vi "SerialWrite&ReadToArduinoLEDBlinkyExample.vi"(8 "error in (no error)":errorcluster, 10 "Text Ring":u16(ring) items=["LED_OFF", "LED_ON"], 11 "ArduinoComPort":refnum<visa-resource-name>) -> (0 "error out":errorcluster, 3 "read buffer":string)   [LabVIEW 2020]
uses:
  <vilib>/Instr/_visa.llb/VISA Configure Serial Port (Instr).vi
panel:
  in  "Send Cmd":bool
  in  "stop":bool
  # "`"
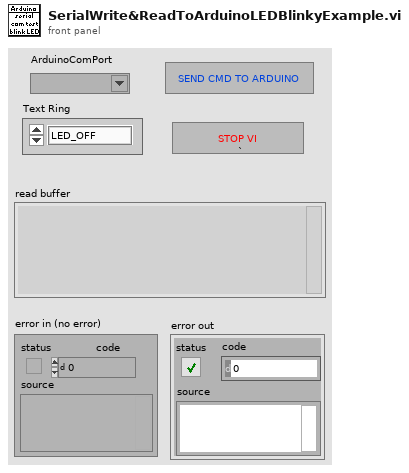
[diagram p1: front panel]
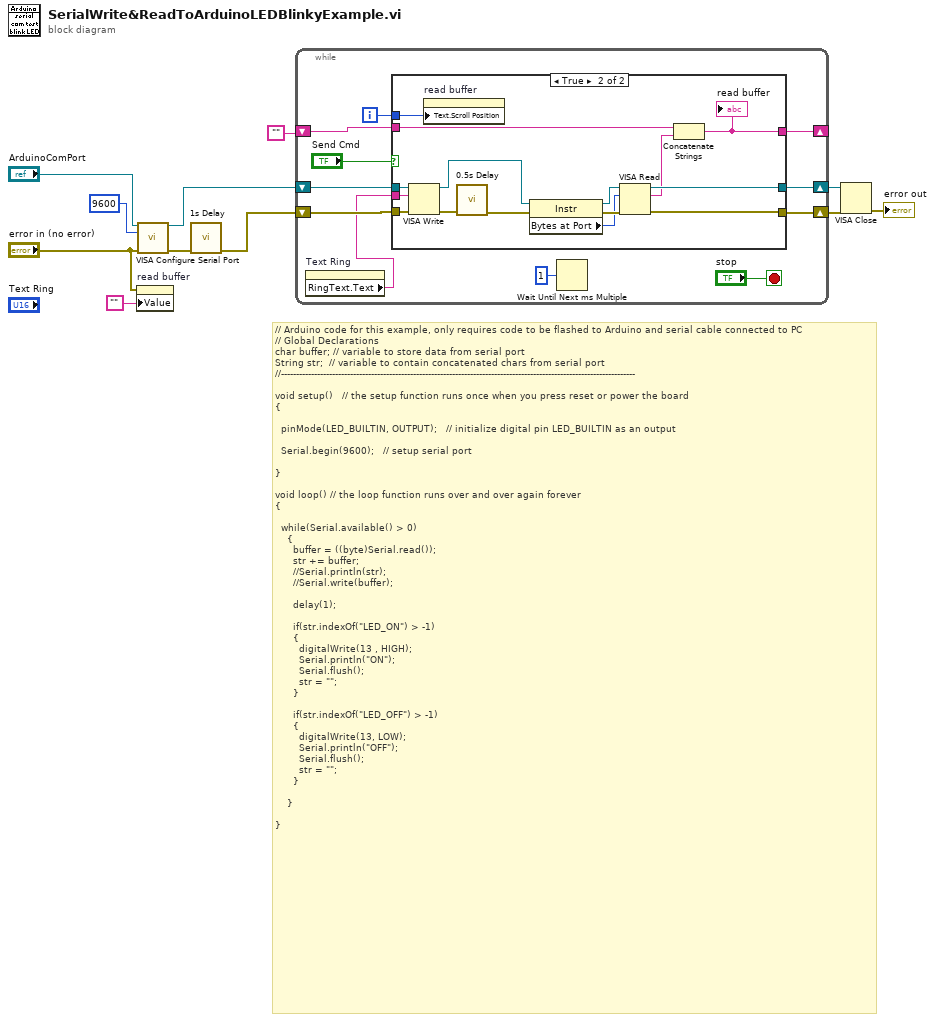
[diagram p0: block diagram]
diagram:
  # "// Arduino code for this example, only requires code to be flashed to Arduino and serial cable connected to PC\n// Global Declarations\nchar buffer; // variable to store data from serial port\nString str;  // variable to contain concatenated chars from serial port\n//----------------------------------------------------------------------------------------------------------------------\n \nvoid setup()   // the setup function runs once when you press reset or power the board \n{\n\n  pinMode(LED_BUILTIN, OUTPUT);   // initialize digital pin LED_BUILTIN as an output\n\n  Serial.begin(9600);   // setup serial port\n\n}\n\nvoid loop() // the loop function runs over and over again forever\n{\n\n  while(Serial.available() > 0)\n    {\n      buffer = ((byte)Serial.read());\n      str += buffer;\n      //Serial.println(str);\n      //Serial.write(buffer);\n\n      delay(1);\n      \n      if(str.indexOf(\"LED_ON\") > -1) \n      {\n        digitalWrite(13 , HIGH);\n        Serial.println(\"ON\");\n        Serial.flush();\n        str = \"\";\n      }\n\n      if(str.indexOf(\"LED_OFF\") > -1)  \n      {\n        digitalWrite(13, LOW);\n        Serial.println(\"OFF\");\n        Serial.flush();\n        str = \"\";\n      }\n\n    }\n\n}"
  n1 = property on="read buffer" class="Str"(error in="error in (no error)", "Value"="") -> ()  [unwired: 1 in, 2 out]
  n2 = call-poly "VISA Configure Serial Port"("VISA resource name"="ArduinoComPort", "baud rate (9600)"=u32 9600, "error in (no error)"="error in (no error)") -> ("VISA resource name out"=w11:refnum<visa-resource-name>, "error out"=w8:errorcluster)  [unwired: 11 in]
  n3 = call "1s Delay"("error in (no error)"=w8) -> ("error out"=w7:errorcluster)  [unwired: 10 in]
  n4 = while {
    shift-right: [w21] -> w5
    shift-left: w7 -> [w20]
    shift-right: [w19] -> _
    shift-left: "" -> [w18]
    shift-right: [w14] -> w3
    shift-left: w11 -> [w22]
    i -> [w13]
    stop <- "stop" stop-if-true
    n5 = property on="Text Ring" class="Ring (strict)"() -> ("RingText.Text"=w12:string)  [unwired: 2 in, 2 out]
    n6 = case shown="True" "Send Cmd" {
      tunnel: w22 -> [w23 w40]
      tunnel: [w24 w30] -> w21
      tunnel: w20 -> [w24 w33]
      tunnel: w12 -> [_ w32]
      tunnel: [w25 w26] -> w19
      tunnel: w18 -> [w25 w31]
      tunnel: [w23 w29] -> w14
      tunnel: w13 -> [_ w28]
      frame False {
      }
      frame True {
        n7 = VISA Write(VISA resource name=w40, write buffer=w32, error in (no error)=w33) -> (VISA resource name out=w37:refnum<visa-resource-name>, error out=w39:errorcluster)  [unwired: 1 out]
        n8 = property on="read buffer" class="Str"("Text.Scroll Position"=w28) -> ()  [unwired: 2 in, 2 out]
        n9 = call "0.5s Delay"("error in (no error)"=w39) -> ("error out"=w38:errorcluster)  [unwired: 10 in]
        n10 = property class="Instr"(reference=w37, error in=w38) -> (reference out=w35:refnum<visa-resource-name>, error out=w36:errorcluster, "Bytes at Port"=w34:u32)
        n11 = VISA Read(VISA resource name=w35, byte count=w34, error in (no error)=w36) -> (VISA resource name out=w29:refnum<visa-resource-name>, read buffer=w27:string, error out=w30:errorcluster)  [unwired: 1 out]
        n12 = Concatenate Strings(w31, w27) -> (w26:string)
        "read buffer" <- w26
      }
    }
    n13 = Wait Until Next ms Multiple(millisecond multiple=u32 1 ("millisecond timer value")) -> ()  [unwired: 1 out]
  }
  n14 = VISA Close(VISA resource name=w3, error in (no error)=w5) -> (error out=→"error out":errorcluster)
